vi "Initialize.vi"(11 "task name":string caption="task name (none)") -> (3 "asset utilization":refnum<class "NI SystemLink Asset Utilization.lvclass">)   [LabVIEW 2019]
uses:
  SupportVIs/NI SystemLink Asset Utilization.lvclass
  SupportVIs/Start Utilization (All).vi
  SupportVIs/Start Utilization (Single).vi
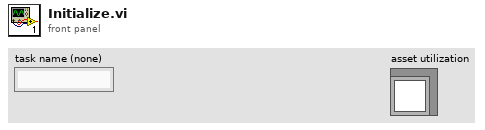
[diagram p1: front panel]
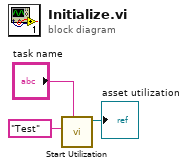
[diagram p0: block diagram]
diagram:
  n1 = call-poly "Start Utilization.vi"("task name"="task name", "utilization category"="Test") -> ("asset utilization"=→"asset utilization":refnum<class "NI SystemLink Asset Utilization.lvclass">)  [unwired: 8 in, 1 out]
